vi "Method Builder.vi"(0 "Input A":T12={"Element A"=0, "Scan Rate A"={"DE (V)"=0.2, "Dt (s)"=1.0}, "Input--Timing A"={"Duration (s)"=30.0, "Sample Rate (ms)"=100.0, "Frequency (mHz)"=1000.0, "Repeat n Times"=0}, "Input--Potential A"={"Ei (V)"=0.0, "Ef (V)"=1.0, "E1 (V)"=1.0, "E2 (V)"=-1.0, "Duty Cycle (%)"=50.0}} {"Scan Rate A"."Dt (s)" format="%0.2f"; "Scan Rate A"."DE (V)" format="%0.2f"; "Element A" items=["Disabled", "Potentiostatic", "Linear Ramp", "Staircase Ramp", "Triangle Wave", "Square Wave", "Staircase Wave", "Sine Wave"]}, 1 "Mode":u16(ring) items=["Sequence: A->B->C->D->E", "Superimpose: A + B"], 2 "Potential Calibration":dbl[][](array[numeric])=[[1.0, 0.0, 5.4592, 5.4592]], 5 "Input B":T11={"Element B"=0, "Input--Potential B"={"Ei (V)"=0.0, "Ef (V)"=1.0, "E1 (V)"=1.0, "E2 (V)"=-1.0, "Duty Cycle (%)"=50.0}, "Input--Timing B"={"Duration (s)"=30.0, "Sample Rate (ms)"=100.0, "Frequency (mHz)"=1000.0, "Repeat n Times"=0}, "Scan Rate B"={"DE (V)"=0.2, "Dt (s)"=1.0}} {"Scan Rate B"."Dt (s)" format="%0.2f"; "Scan Rate B"."DE (V)" format="%0.2f"; "Element B" items=["Disabled", "Potentiostatic", "Linear Ramp", "Staircase Ramp", "Triangle Wave", "Square Wave", "Staircase Wave", "Sine Wave"]}, 7 "Input C":T10={"Scan Rate C"={"DE (V)"=0.2, "Dt (s)"=1.0}, "Input--Timing C"={"Duration (s)"=30.0, "Sample Rate (ms)"=100.0, "Frequency (mHz)"=1000.0, "Repeat n Times"=0}, "Input--Potential C"={"Ei (V)"=0.0, "Ef (V)"=1.0, "E1 (V)"=1.0, "E2 (V)"=-1.0, "Duty Cycle (%)"=50.0}, "Element C"=0} {"Scan Rate C"."Dt (s)" format="%0.2f"; "Scan Rate C"."DE (V)" format="%0.2f"; "Element C" items=["Disabled", "Potentiostatic", "Linear Ramp", "Staircase Ramp", "Triangle Wave", "Square Wave", "Staircase Wave", "Sine Wave"]}, 9 "Input D":T9={"Scan Rate D"={"DE (V)"=0.2, "Dt (s)"=1.0}, "Input--Timing D"={"Duration (s)"=30.0, "Sample Rate (ms)"=100.0, "Frequency (mHz)"=1000.0, "Repeat n Times"=0}, "Input--Potential D"={"Ei (V)"=0.0, "Ef (V)"=1.0, "E1 (V)"=1.0, "E2 (V)"=-1.0, "Duty Cycle (%)"=50.0}, "Element D"=0} {"Scan Rate D"."Dt (s)" format="%0.2f"; "Scan Rate D"."DE (V)" format="%0.2f"; "Element D" items=["Disabled", "Potentiostatic", "Linear Ramp", "Staircase Ramp", "Triangle Wave", "Square Wave", "Staircase Wave", "Sine Wave"]}, 11 "Input E":T8={"Scan Rate E"={"DE (V)"=0.2, "Dt (s)"=1.0}, "Input--Timing E"={"Duration (s)"=30.0, "Sample Rate (ms)"=100.0, "Frequency (mHz)"=1000.0, "Repeat n Times"=0}, "Input--Potential E"={"Ei (V)"=0.0, "Ef (V)"=1.0, "E1 (V)"=1.0, "E2 (V)"=-1.0, "Duty Cycle (%)"=50.0}, "Element E"=0} {"Scan Rate E"."Dt (s)" format="%0.2f"; "Scan Rate E"."DE (V)" format="%0.2f"; "Element E" items=["Disabled", "Potentiostatic", "Linear Ramp", "Staircase Ramp", "Triangle Wave", "Square Wave", "Staircase Wave", "Sine Wave"]}, 12 "Cycles":i32=1, 13 "Arduino In":cluster{"Error In":errorcluster, "LINX In":T2}) -> (4 "Output":T1, 10 "Preview (Single Cycle)":cluster{dbl[], "Preview":dbl[]}[](graph), 14 "Arduino Out":cluster{"Error Out":errorcluster, "LINX Out":T2}, 15 "Signal Frequencies (mHz)":cluster{"A":dbl, "B":dbl})   [LabVIEW 2022 SP3]
uses:
  <vilib>/MakerHub/LINX/Private/Type Defs/LINX Ref.ctl
  <vilib>/MakerHub/LINX/Private/Type Defs/Platform.ctl
  <vilib>/MakerHub/LINX/Private/Type Defs/Interface.ctl
  <vilib>/MakerHub/LINX/Private/Device/Type Defs/LINX Device Config.ctl
  <vilib>/MakerHub/LINX/Private/Device/Type Defs/TCP Config.ctl
  <vilib>/MakerHub/LINX/Private/Device/Type Defs/Channels.ctl
  <vilib>/MakerHub/LINX/LMH-LINX.lvlib
  <vilib>/MakerHub/LINX/Private/Device/Device.lvlib
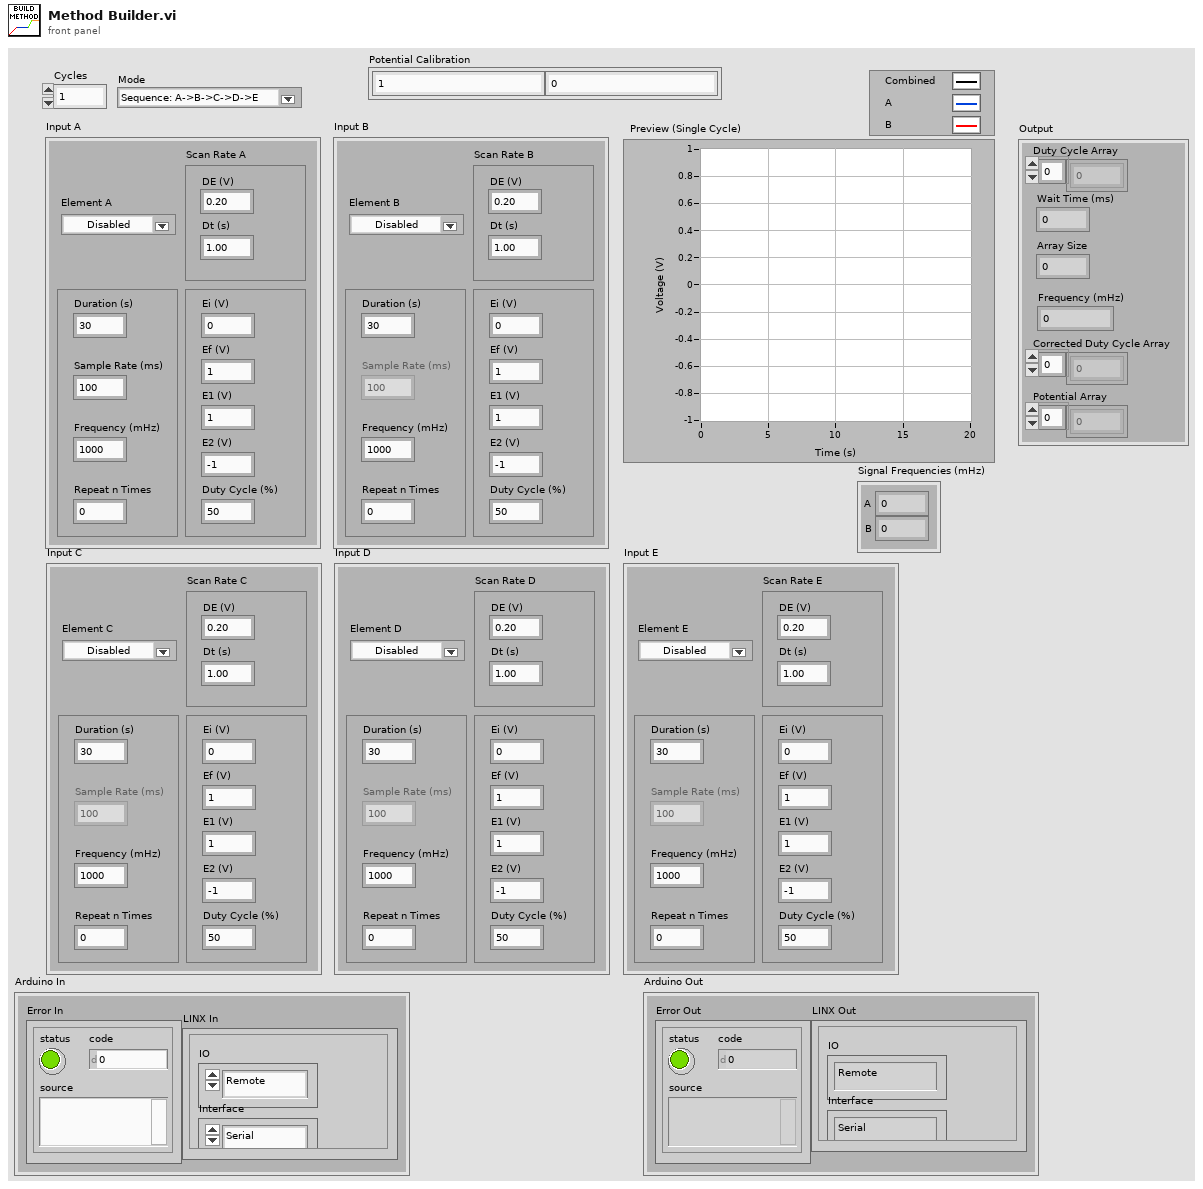
[diagram p1: front panel]
types:
  T1 = cluster{"Duty Cycle Array":dbl[], "Wait Time (ms)":dbl, "Array Size":i32, "Frequency (mHz)":dbl, "Corrected Duty Cycle Array":dbl[], "Potential Array":dbl[]}
  T2 = typedef "LMH-LINX.lvlib/LINX Ref.ctl" = cluster{"IO":T3, "Interface":T4, "LINX Device Config":T5}
  T3 = typedef "LMH-LINX.lvlib/Platform.ctl" = enum16{"Remote", "Local"}
  T4 = typedef "LMH-LINX.lvlib/Interface.ctl" = enum16{"Serial", "TCP"}
  T5 = typedef "LMH-LINX.lvlib/Device.lvlib/LINX Device Config.ctl" = cluster{"Interface":T4, "COM Port":refnum<visa-resource-name>, "TCP Configuration":T6, "Device Family":u8, "Device ID":u8, "Device Name":string, "TCP Ref":refnum<k5>, "Channels":T7}
  T6 = typedef "LMH-LINX.lvlib/Device.lvlib/TCP Config.ctl" = cluster{"IP Address":string, "Port":u16}
  T7 = typedef "LMH-LINX.lvlib/Channels.ctl" = cluster{"DI":u8[], "DO":u8[], "AI":u8[], "AO":u8[], "PWM":u8[], "QE":u8[], "UART":u8[], "I2C 2":u8[], "SPI":u8[], "CAN":u8[], "Servo":u8[], "AI Ref (V)":dbl, "AI Resolution (Bits)":u8, "AO Ref (V)":dbl, "AO Resolution (Bits)":u8}
  T8 = cluster{"Scan Rate E":cluster{"DE (V)":dbl, "Dt (s)":dbl}, "Input--Timing E":cluster{"Duration (s)":dbl, "Sample Rate (ms)":dbl, "Frequency (mHz)":dbl, "Repeat n Times":i32}, "Input--Potential E":cluster{"Ei (V)":dbl, "Ef (V)":dbl, "E1 (V)":dbl, "E2 (V)":dbl, "Duty Cycle (%)":dbl}, "Element E":u16}
  T9 = cluster{"Scan Rate D":cluster{"DE (V)":dbl, "Dt (s)":dbl}, "Input--Timing D":cluster{"Duration (s)":dbl, "Sample Rate (ms)":dbl, "Frequency (mHz)":dbl, "Repeat n Times":i32}, "Input--Potential D":cluster{"Ei (V)":dbl, "Ef (V)":dbl, "E1 (V)":dbl, "E2 (V)":dbl, "Duty Cycle (%)":dbl}, "Element D":u16}
  T10 = cluster{"Scan Rate C":cluster{"DE (V)":dbl, "Dt (s)":dbl}, "Input--Timing C":cluster{"Duration (s)":dbl, "Sample Rate (ms)":dbl, "Frequency (mHz)":dbl, "Repeat n Times":i32}, "Input--Potential C":cluster{"Ei (V)":dbl, "Ef (V)":dbl, "E1 (V)":dbl, "E2 (V)":dbl, "Duty Cycle (%)":dbl}, "Element C":u16}
  T11 = cluster{"Element B":u16, "Input--Potential B":cluster{"Ei (V)":dbl, "Ef (V)":dbl, "E1 (V)":dbl, "E2 (V)":dbl, "Duty Cycle (%)":dbl}, "Input--Timing B":cluster{"Duration (s)":dbl, "Sample Rate (ms)":dbl, "Frequency (mHz)":dbl, "Repeat n Times":i32}, "Scan Rate B":cluster{"DE (V)":dbl, "Dt (s)":dbl}}
  T12 = cluster{"Element A":u16, "Scan Rate A":cluster{"DE (V)":dbl, "Dt (s)":dbl}, "Input--Timing A":cluster{"Duration (s)":dbl, "Sample Rate (ms)":dbl, "Frequency (mHz)":dbl, "Repeat n Times":i32}, "Input--Potential A":cluster{"Ei (V)":dbl, "Ef (V)":dbl, "E1 (V)":dbl, "E2 (V)":dbl, "Duty Cycle (%)":dbl}}
  T13 = cluster{"Ei (V)":dbl, "Ef (V)":dbl, "E1 (V)":dbl, "E2 (V)":dbl, "Duty Cycle (%)":dbl}
  T14 = cluster{"Duration (s)":dbl, "Sample Rate (ms)":dbl, "Frequency (mHz)":dbl, "Repeat n Times":i32}
  T15 = cluster{"Frequency (mHz)":dbl, "Frequency (mHz)":dbl}
  T16 = cluster{dbl[], "Wait Time (ms)":dbl, i32, "Frequency (mHz)":dbl, dbl[], dbl[]}
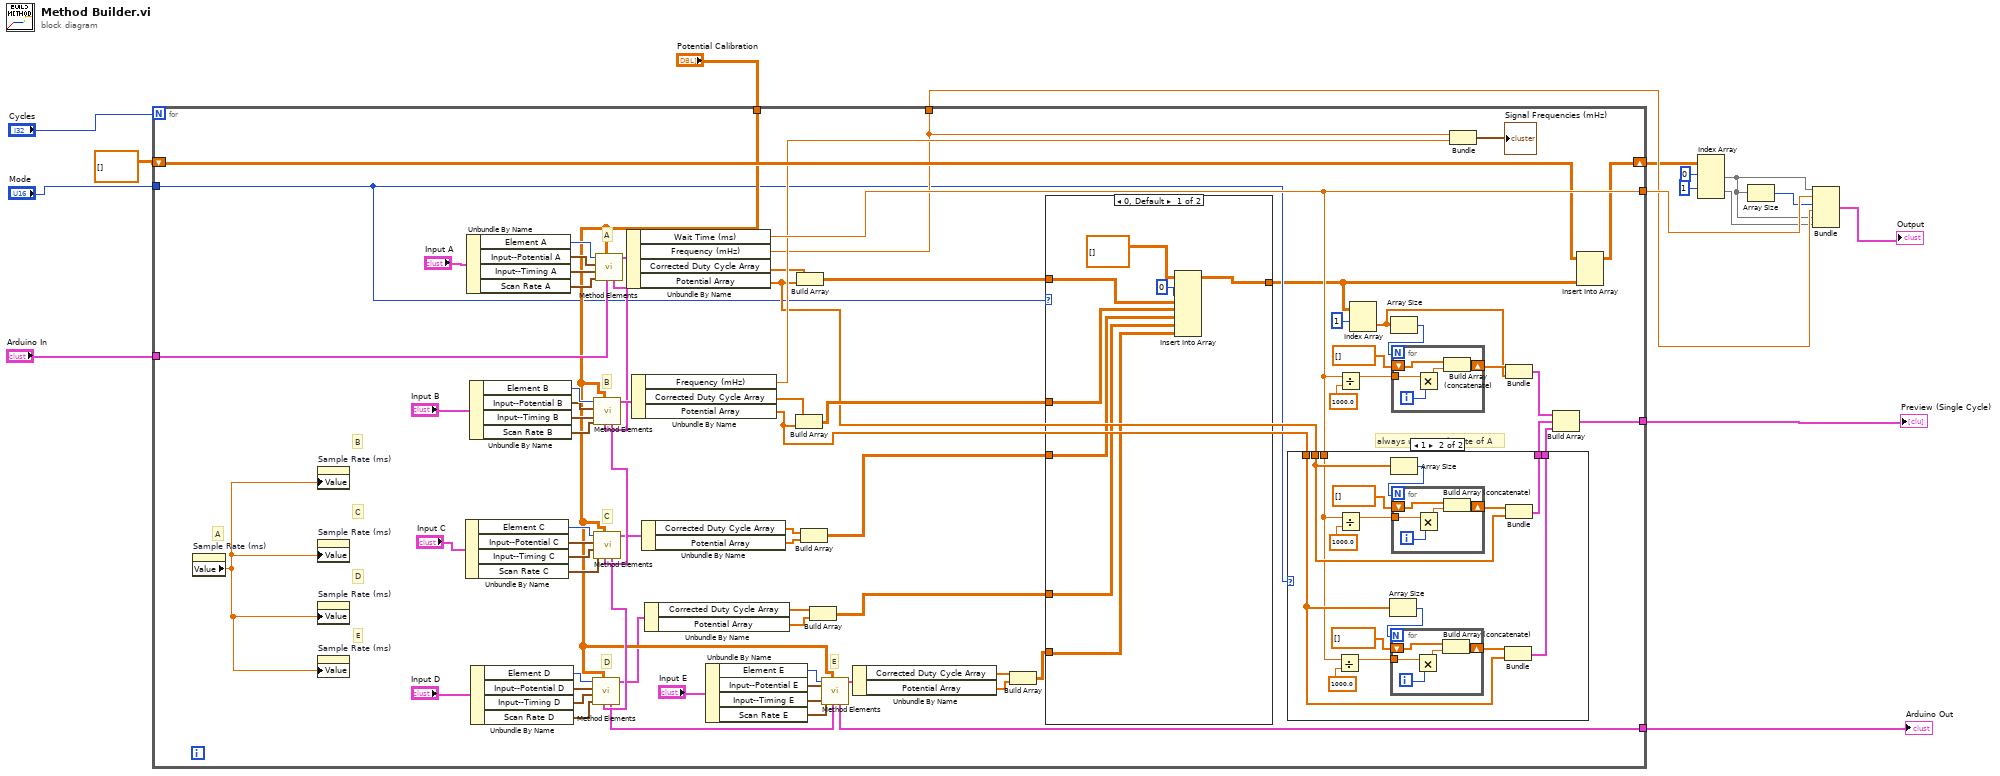
[diagram p0: block diagram]
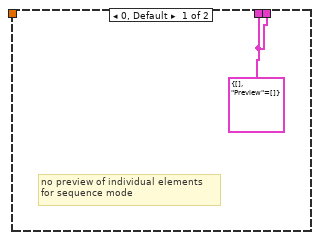
[diagram p2: hidden frame]
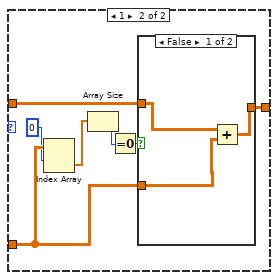
[diagram p3: hidden frame]
diagram:
  n1 = for {
    N: "Cycles" -> [_]
    tunnel: "Mode" -> [w32]
    tunnel: [w79] -> w11
    tunnel: [w78] -> w14
    shift-right: [w76] -> w5
    shift-left: dbl[][] [] -> [w77]
    tunnel: "Arduino In" -> [w48]
    tunnel: [w43] -> w12
    tunnel: [w42] -> w9
    tunnel: "Potential Calibration" -> [w40]
    # "A"
    # "E"
    # "D"
    # "C"
    # "B"
    # "E"
    # "D"
    # "C"
    # "always use sample rate of A"
    # "B"
    # "A"
    n2 = property on="Sample Rate (ms)" class="DigNum (strict)"() -> ("Value"=w41:dbl)  [unwired: 2 in, 2 out]
    n3 = property on="Sample Rate (ms)" class="DigNum (strict)"("Value"=w41) -> ()  [unwired: 2 in, 2 out]
    n4 = property on="Sample Rate (ms)" class="DigNum (strict)"("Value"=w41) -> ()  [unwired: 2 in, 2 out]
    n5 = property on="Sample Rate (ms)" class="DigNum (strict)"("Value"=w41) -> ()  [unwired: 2 in, 2 out]
    n6 = property on="Sample Rate (ms)" class="DigNum (strict)"("Value"=w41) -> ()  [unwired: 2 in, 2 out]
    n7 = Unbundle By Name("Input C") -> ("Element C"=w65:u16, "Input--Potential C"=w64:T13, "Input--Timing C"=w63:T14, "Scan Rate C"=w62:cluster{"DE (V)":dbl, "Dt (s)":dbl})
    n8 = Unbundle By Name("Input A") -> ("Element A"=w74:u16, "Input--Potential A"=w73:T13, "Input--Timing A"=w72:T14, "Scan Rate A"=w71:cluster{"DE (V)":dbl, "Dt (s)":dbl})
    n9 = Unbundle By Name("Input B") -> ("Element B"=w70:u16, "Input--Potential B"=w69:T13, "Input--Timing B"=w68:T14, "Scan Rate B"=w67:cluster{"DE (V)":dbl, "Dt (s)":dbl})
    n10 = Unbundle By Name("Input D") -> ("Element D"=w60:u16, "Input--Potential D"=w59:T13, "Input--Timing D"=w58:T14, "Scan Rate D"=w57:cluster{"DE (V)":dbl, "Dt (s)":dbl})
    n11 = call "Method Elements.vi"("Arduino In"=w48, "Potential Calibration"=w40, "Input--Scan Rate"=w71, "Input--Timing"=w72, "Input--Potential"=w73, "Element"=w74) -> ("Output"=w88:T1, "Arduino Out"=w47:cluster{"Error Out":errorcluster, "LINX Out":T2})  [unwired: 4 in]
    n12 = call "Method Elements.vi"("Arduino In"=w47, "Potential Calibration"=w40, "Input--Scan Rate"=w67, "Input--Timing"=w68, "Input--Potential"=w69, "Element"=w70) -> ("Output"=w87:T1, "Arduino Out"=w46:cluster{"Error Out":errorcluster, "LINX Out":T2})  [unwired: 4 in]
    n13 = call "Method Elements.vi"("Arduino In"=w46, "Potential Calibration"=w40, "Input--Scan Rate"=w62, "Input--Timing"=w63, "Input--Potential"=w64, "Element"=w65) -> ("Output"=w30:T1, "Arduino Out"=w45:cluster{"Error Out":errorcluster, "LINX Out":T2})  [unwired: 4 in]
    n14 = call "Method Elements.vi"("Arduino In"=w45, "Potential Calibration"=w40, "Input--Scan Rate"=w57, "Input--Timing"=w58, "Input--Potential"=w59, "Element"=w60) -> ("Output"=w26:T1, "Arduino Out"=w44:cluster{"Error Out":errorcluster, "LINX Out":T2})  [unwired: 4 in]
    n15 = Unbundle By Name(w88) -> ("Wait Time (ms)"=w79:dbl, "Frequency (mHz)"=w42:dbl, "Corrected Duty Cycle Array"=w34:dbl[], "Potential Array"=w35:dbl[])
    n16 = Unbundle By Name(w87) -> ("Frequency (mHz)"=w49:dbl, "Corrected Duty Cycle Array"=w38:dbl[], "Potential Array"=w33:dbl[])
    n17 = Unbundle By Name(w30) -> ("Corrected Duty Cycle Array"=w28:dbl[], "Potential Array"=w29:dbl[])
    n18 = Unbundle By Name(w26) -> ("Corrected Duty Cycle Array"=w25:dbl[], "Potential Array"=w24:dbl[])
    n19 = Unbundle By Name("Input E") -> ("Element E"=w55:u16, "Input--Potential E"=w54:T13, "Input--Timing E"=w53:T14, "Scan Rate E"=w52:cluster{"DE (V)":dbl, "Dt (s)":dbl})
    n20 = Build Array(w38, w33) -> (w37:dbl[][])
    n21 = Build Array(w34, w35) -> (w39:dbl[][])
    n22 = Build Array(w28, w29) -> (w27:dbl[][])
    n23 = Build Array(w25, w24) -> (w23:dbl[][])
    n24 = call "Method Elements.vi"("Arduino In"=w44, "Potential Calibration"=w40, "Input--Scan Rate"=w52, "Input--Timing"=w53, "Input--Potential"=w54, "Element"=w55) -> ("Output"=w22:T1, "Arduino Out"=w43:cluster{"Error Out":errorcluster, "LINX Out":T2})  [unwired: 4 in]
    n25 = Unbundle By Name(w22) -> ("Corrected Duty Cycle Array"=w21:dbl[], "Potential Array"=w20:dbl[])
    n26 = Build Array(w21, w20) -> (w19:dbl[][])
    n27 = case shown="0, Default" w32 {
      tunnel: w27 -> [w123 _]
      tunnel: w23 -> [w124 _]
      tunnel: w19 -> [w125 _]
      tunnel: w39 -> [w121 w132]
      tunnel: w37 -> [w122 w131]
      tunnel: [w127 w128] -> w17
      frame 0, Default {
        n28 = Insert Into Array(array=dbl[][] [], index (col)=0 ("disabled index (col)"), new element #1=w121, new element #2=w122, new element #3=w123, new element #4=w124, new element #5=w125) -> (w127:dbl[][])  [unwired: 1 in]
      }
      frame 1 {
        n29 = Index Array(array=w131, index (row)=0) -> (element=w129:dbl[])  [unwired: 1 in]
        n30 = Array Size(array=w129) -> (size(s)=w133:i32)
        n31 = Equal To 0?(x=w133) -> (x = 0?=w134:bool)
        n32 = case shown="False" w134 {
          tunnel: w132 -> [w136 w138]
          tunnel: w131 -> [w137 _]
          tunnel: [w135 w138] -> w128
          frame False {
            n33 = Add(x=w136, y=w137) -> (x+y=w135:dbl[][])
          }
          frame True {
            # "if B is disabled, no\nsuperposition takes\nplace"
          }
        }
      }
    }
    n34 = case shown="1" w32 {
      tunnel: w35 -> [_ w99]
      tunnel: [w89 w98] -> w81
      tunnel: w33 -> [_ w92]
      tunnel: w79 -> [_ w91]
      tunnel: [w89 w90] -> w80
      frame 0, Default {
        w89 = cluster{dbl[], "Preview":dbl[]} {[], "Preview"=[]}
        # "no preview of individual elements\nfor sequence mode"
      }
      frame 1 {
        n35 = Divide(x=w91, y=1000.0) -> (x/y=w94:dbl)
        n36 = Divide(x=w91, y=1000.0) -> (x/y=w103:dbl)
        n37 = Array Size(array=w92) -> (size(s)=w93:i32)
        n38 = Array Size(array=w99) -> (size(s)=w104:i32)
        n39 = for {
          N: w93 -> [_]
          tunnel: w94 -> [w108]
          shift-right: [w106] -> w97
          shift-left: dbl[] [] -> [w105]
          i -> [w109]
          n40 = Multiply(x=w108, y=w109) -> (x*y=w107:dbl)
          n41 = Build Array (concatenate)(w105, w107) -> (w106:dbl[])
        }
        n42 = for {
          N: w104 -> [_]
          tunnel: w103 -> [w113]
          shift-right: [w111] -> w100
          shift-left: dbl[] [] -> [w110]
          i -> [w114]
          n43 = Multiply(x=w113, y=w114) -> (x*y=w112:dbl)
          n44 = Build Array (concatenate)(w110, w112) -> (w111:dbl[])
        }
        n45 = Bundle(w97, "Potential Array"=w92) -> (w90:cluster{dbl[], "Potential Array":dbl[]})  [unwired: 1 in]
        n46 = Bundle(w100, "Potential Array"=w99) -> (w98:cluster{dbl[], "Potential Array":dbl[]})  [unwired: 1 in]
      }
    }
    n47 = Divide(x=w79, y=1000.0) -> (x/y=w85:dbl)
    n48 = Index Array(array=w17, index (row)=1) -> (element=w18:dbl[])  [unwired: 1 in]
    n49 = Array Size(array=w18) -> (size(s)=w86:i32)
    n50 = for {
      N: w86 -> [_]
      tunnel: w85 -> [w118]
      shift-right: [w116] -> w83
      shift-left: dbl[] [] -> [w115]
      i -> [w119]
      n51 = Multiply(x=w118, y=w119) -> (x*y=w117:dbl)
      n52 = Build Array (concatenate)(w115, w117) -> (w116:dbl[])
    }
    n53 = Bundle("Frequency (mHz)"=w42, "Frequency (mHz)"=w49) -> (→"Signal Frequencies (mHz)":T15)  [unwired: 1 in]
    n54 = Bundle(w83, "array"=w18) -> (w82:cluster{dbl[], "array":dbl[]})  [unwired: 1 in]
    n55 = Build Array(w82, w81, w80) -> (w78:cluster{dbl[], "Potential Array":dbl[]}[])
    n56 = Insert Into Array(array=w77, new element=w17) -> (w76:dbl[][])  [unwired: 2 in]
  }
  "Preview (Single Cycle)" <- w14
  "Arduino Out" <- w12
  n57 = Index Array(array=w5, index (row) #1=0 ("index (row)"), index (row) #2=1 ("index (row)")) -> (element #1=w2:dbl[], element #2=w1:dbl[])  [unwired: 2 in]
  n58 = Array Size(array=w2) -> (size(s)=w10:i32)
  n59 = Bundle(w2, "Wait Time (ms)"=w11, w10, "Frequency (mHz)"=w9, w2, w1) -> (→"Output":T16)  [unwired: 1 in]
